vi "Ohmmeter.vi"() -> ()   [LabVIEW 2020]
uses:
  <vilib>/MakerHub/LINX/Private/Type Defs/LINX Ref.ctl
  <vilib>/MakerHub/LINX/Private/Type Defs/Platform.ctl
  <vilib>/MakerHub/LINX/Private/Type Defs/Interface.ctl
  <vilib>/MakerHub/LINX/Private/Device/Type Defs/LINX Device Config.ctl
  <vilib>/MakerHub/LINX/Private/Device/Type Defs/TCP Config.ctl
  <vilib>/MakerHub/LINX/Private/Device/Type Defs/Channels.ctl
  <vilib>/MakerHub/LINX/Public/Peripherals/Analog/Analog Read 1 Chan.vi
  <vilib>/MakerHub/LINX/Public/Peripherals/Analog/Analog Read N Chans.vi
  <vilib>/MakerHub/LINX/Private/Local IO/LinxAnalogRead.vi
  <vilib>/MakerHub/LINX/Public/Utilities/Check Channel.vi
  <vilib>/MakerHub/LINX/Public/Utilities/Open Serial.vi
  <vilib>/MakerHub/LINX/Private/Utilties/Generate Error.vi
  <vilib>/MakerHub/LINX/LMH-LINX.lvlib
  <vilib>/MakerHub/LINX/Private/Device/Device.lvlib
panel:
  in  "Tab Control":enum32{"Serial Com.", "Circuit", "Readings"}(tab)
  in  "Serial Port":refnum<visa-resource-name>="N/A"
  out "Connected?":bool
  in  "Start Serial Communication":bool
  in  "Stop Serial \nCommunication":bool
  out "Device Name":string
  out "2D Picture":picture
  in  "Ohmmeter Circuit\nParameters":T1
  in  "Read Data":bool
  in  "Pause Readings":bool
  in  "Save Data":bool
  out "Data History":dbl(graph)
  out "Reading?":bool
  in  "Read Freq. (Hz)":dbl
  in  "Stop Application":bool
  # "Serial Ohmmeter V.I."
  # "Serial  Communication"
  # "Communication State"
  # "Circuit  Parameters"
  # "Circuit Schematics"
  # "Readings State"
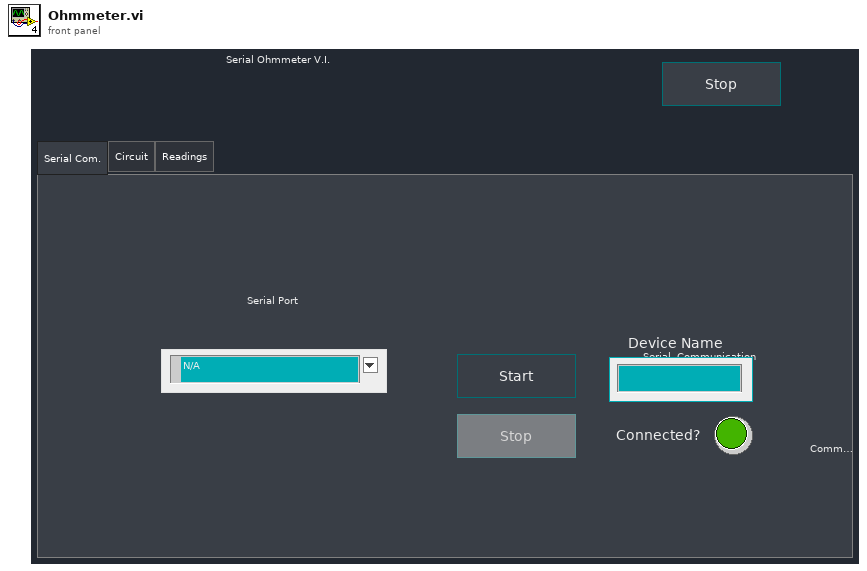
[diagram p1: front panel]
types:
  T1 = cluster{" Circuit Total Voltage (V)":dbl, " Reference Resistor (W)":dbl, "Analog Pin":u8}
  T2 = typedef "LMH-LINX.lvlib/LINX Ref.ctl" = cluster{"IO":T3, "Interface":T4, "LINX Device Config":T5}
  T3 = typedef "LMH-LINX.lvlib/Platform.ctl" = enum16{"Remote", "Local"}
  T4 = typedef "LMH-LINX.lvlib/Interface.ctl" = enum16{"Serial", "TCP"}
  T5 = typedef "LMH-LINX.lvlib/Device.lvlib/LINX Device Config.ctl" = cluster{"Interface":T4, "COM Port":refnum<visa-resource-name>, "TCP Configuration":T6, "Device Family":u8, "Device ID":u8, "Device Name":string, "TCP Ref":refnum<k5>, "Channels":T7}
  T6 = typedef "LMH-LINX.lvlib/Device.lvlib/TCP Config.ctl" = cluster{"IP Address":string, "Port":u16}
  T7 = typedef "LMH-LINX.lvlib/Channels.ctl" = cluster{"DI":u8[], "DO":u8[], "AI":u8[], "AO":u8[], "PWM":u8[], "QE":u8[], "UART":u8[], "I2C 2":u8[], "SPI":u8[], "CAN":u8[], "Servo":u8[], "AI Ref (V)":dbl, "AI Resolution (Bits)":u8, "AO Ref (V)":dbl, "AO Resolution (Bits)":u8}
  T8 = enum8{"Enabled", "Disabled", "Disabled and Grayed Out"}
  T9 = typedef "imagedata.ctl" = cluster{"image type":i32, "image depth":i32, "image":u8[], "mask":u8[], "colors":u32[], "Rectangle":cluster{"left":i16, "top":i16, "right":i16, "bottom":i16}}
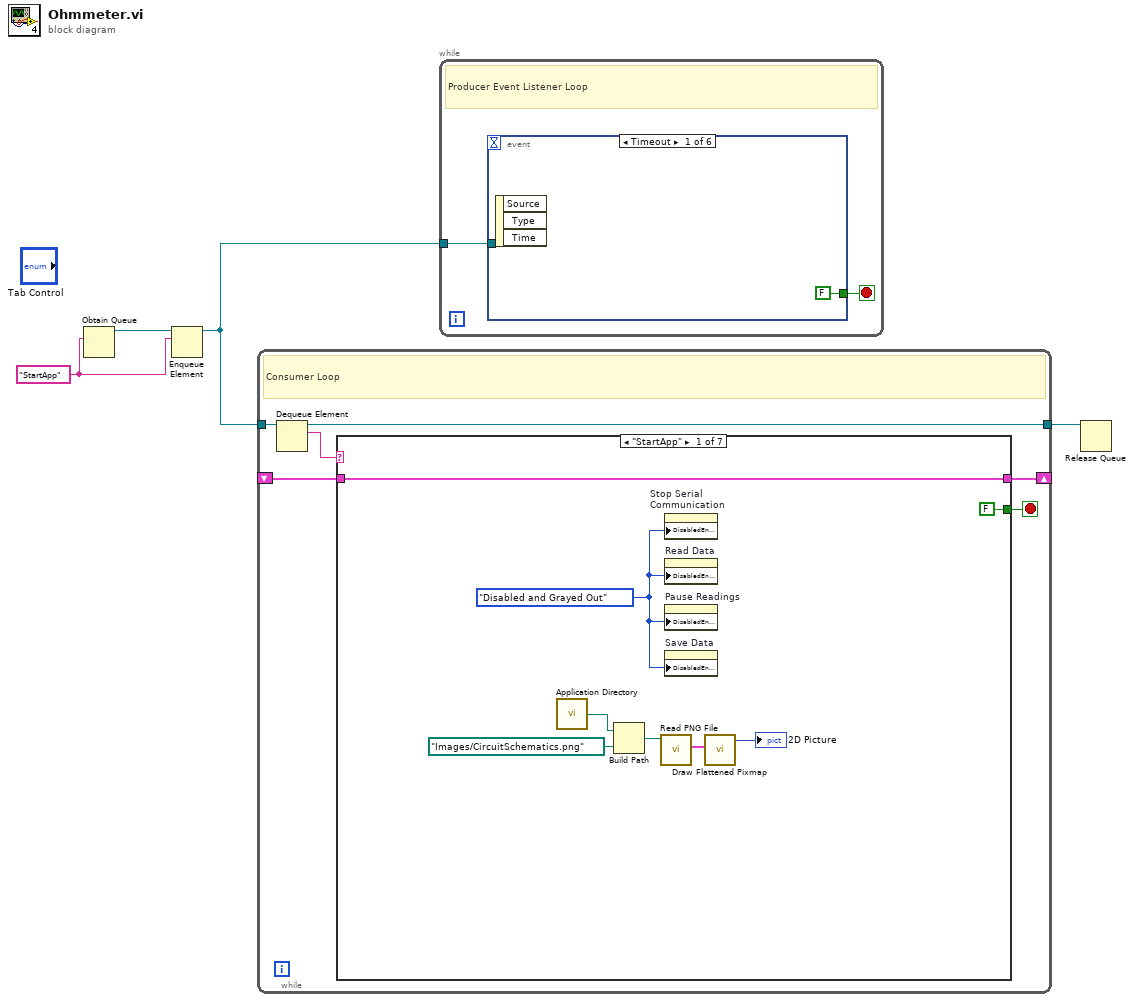
[diagram p0: block diagram]
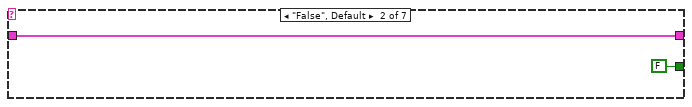
[diagram p2: hidden frame]
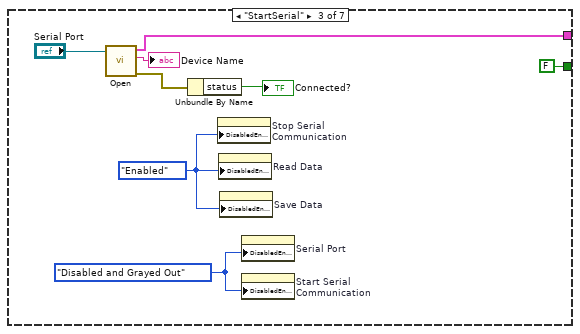
[diagram p3: hidden frame]
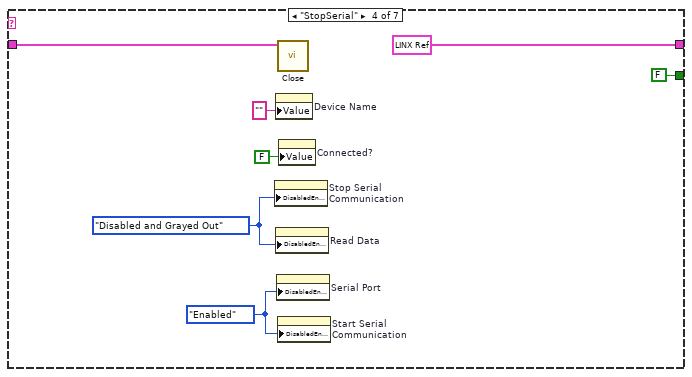
[diagram p4: hidden frame]
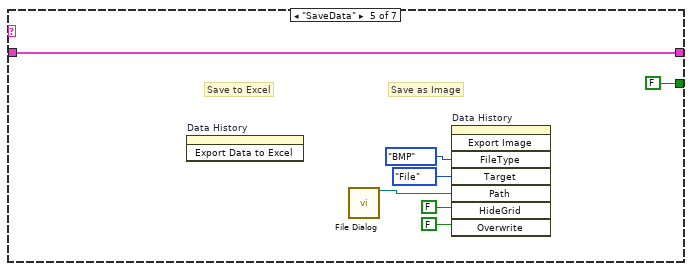
[diagram p5: hidden frame]
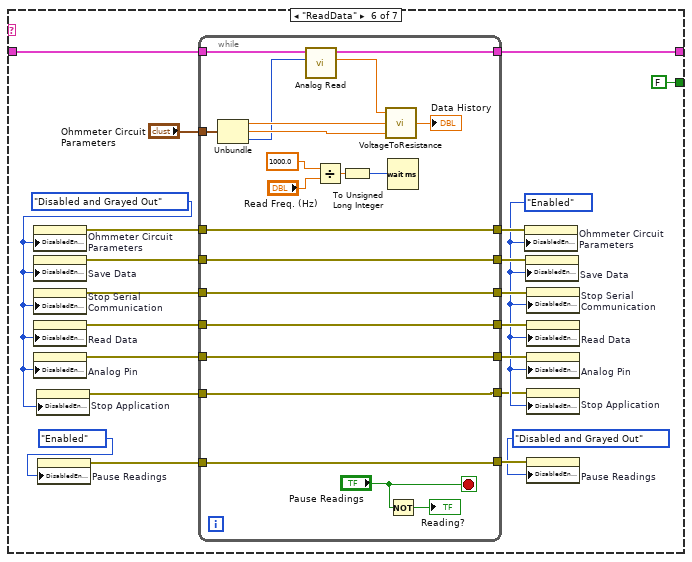
[diagram p6: hidden frame]
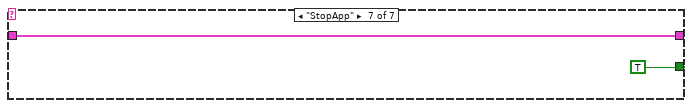
[diagram p7: hidden frame]
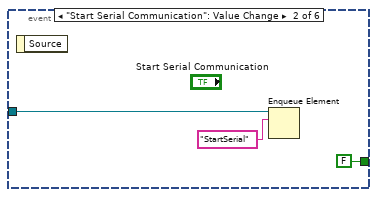
[diagram p8: hidden frame]
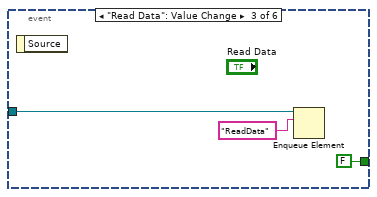
[diagram p9: hidden frame]
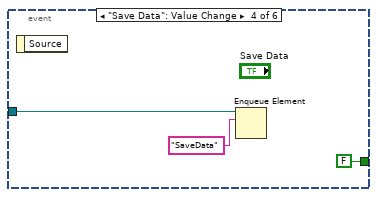
[diagram p10: hidden frame]
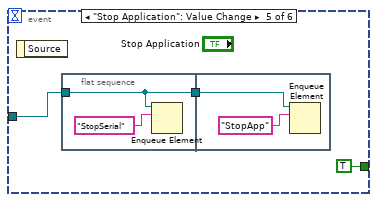
[diagram p11: hidden frame]
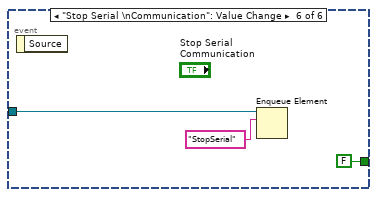
[diagram p12: hidden frame]
diagram:
  w1 = "StartApp"
  n1 = Obtain Queue(element data type=w1) -> (queue out=w2:refnum<queue>)  [unwired: 4 in, 2 out]
  n2 = Enqueue Element(queue=w2, element=w1) -> (queue out=w3:refnum<queue>)  [unwired: 2 in, 2 out]
  n3 = while {
    tunnel: w3 -> [w10]
    tunnel: [w7] -> w4
    shift-right: [w6] -> _
    shift-left: _ -> [w5]
    stop <- w8 stop-if-true
    # "Consumer Loop"
    n4 = Dequeue Element(queue=w10) -> (queue out=w7:refnum<queue>, element=w9:string)  [unwired: 2 in, 2 out]
    n5 = case shown="\"StartApp\"" w9 {
      tunnel: [FALSE FALSE FALSE FALSE FALSE FALSE TRUE] -> w8
      tunnel: [w16 w20 w26 T2 {"IO"=enum."Remote", "Interface"=enum."Serial", "LINX Device Config"={"Interface"=enum."Serial", "COM Port"="", "TCP Configuration"={"IP Address"="", "Port"=0}, "Device Family"=0, "Device ID"=0, "Device Name"="", "TCP Ref"=refnum, "Channels"={"DI"=[], "DO"=[], "AI"=[], "AO"=[], "PWM"=[], "QE"=[], "UART"=[], "I2C 2"=[], "SPI"=[], "CAN"=[], "Servo"=[], "AI Ref (V)"=0.0, "AI Resolution (Bits)"=0, "AO Ref (V)"=0.0, "AO Resolution (Bits)"=0}}} ("LINX Resource") w36 w62 w86] -> w6
      tunnel: w5 -> [w16 w20 _ w35 w36 w64 w86]
      frame "StartApp" {
        w18 = T8."Disabled and Grayed Out" ("Disabled")
        n6 = call <vilib>:"Application Directory.vi"() -> ("Application Directory"=w11:path)
        n7 = Build Path(base path=w11, name or relative path=path "Images/CircuitSchematics.png") -> (appended path=w14:path)
        n8 = call <vilib>:"Read PNG File.vi"("path to PNG file"=w14) -> ("image data"=w13:T9)  [unwired: 8 in, 2 out]
        n9 = property on="Stop Serial \nCommunication" class="Bool"("DisabledEnum"=w18) -> ()  [unwired: 2 in, 2 out]
        n10 = property on="Read Data" class="Bool"("DisabledEnum"=w18) -> ()  [unwired: 2 in, 2 out]
        n11 = property on="Pause Readings" class="Bool"("DisabledEnum"=w18) -> ()  [unwired: 2 in, 2 out]
        n12 = property on="Save Data" class="Bool"("DisabledEnum"=w18) -> ()  [unwired: 2 in, 2 out]
        n13 = call <vilib>:"Draw Flattened Pixmap.vi"("image data"=w13) -> ("new picture"=→"2D Picture":picture)  [unwired: 8 in]
      }
      frame "False", Default {
      }
      frame "StartSerial" {
        w22 = T8."Disabled and Grayed Out" ("Disabled")
        w23 = T8."Enabled" ("Disabled")
        n14 = call-poly <vilib>:"Open.vi"("Serial Port"="Serial Port") -> ("Error Out"=w25:errorcluster, "Device Name"=→"Device Name":string, "LINX Resource"=w26:T2)  [unwired: 8 in]
        n15 = Unbundle By Name(w25) -> ("status"=→"Connected?":bool)
        n16 = property on="Stop Serial \nCommunication" class="Bool"("DisabledEnum"=w23) -> ()  [unwired: 2 in, 2 out]
        n17 = property on="Read Data" class="Bool"("DisabledEnum"=w23) -> ()  [unwired: 2 in, 2 out]
        n18 = property on="Save Data" class="Bool"("DisabledEnum"=w23) -> ()  [unwired: 2 in, 2 out]
        n19 = property on="Serial Port" class="VISAName"("DisabledEnum"=w22) -> ()  [unwired: 2 in, 2 out]
        n20 = property on="Start Serial \nCommunication" class="Bool"("DisabledEnum"=w22) -> ()  [unwired: 2 in, 2 out]
      }
      frame "StopSerial" {
        w31 = T8."Enabled" ("Disabled")
        w30 = T8."Disabled and Grayed Out" ("Disabled")
        n21 = property on="Stop Serial \nCommunication" class="Bool"("DisabledEnum"=w30) -> ()  [unwired: 2 in, 2 out]
        n22 = property on="Device Name" class="Str"("Value"="" ("Device Name")) -> ()  [unwired: 2 in, 2 out]
        n23 = property on="Read Data" class="Bool"("DisabledEnum"=w30) -> ()  [unwired: 2 in, 2 out]
        n24 = property on="Serial Port" class="VISAName"("DisabledEnum"=w31) -> ()  [unwired: 2 in, 2 out]
        n25 = call <vilib>:"Close.vi"("LINX Resource"=w35) -> ()  [unwired: 10 in, 1 out]
        n26 = property on="Start Serial \nCommunication" class="Bool"("DisabledEnum"=w31) -> ()  [unwired: 2 in, 2 out]
        n27 = property on="Connected?" class="Bool (strict)"("Value"=FALSE ("Connected?")) -> ()  [unwired: 2 in, 2 out]
      }
      frame "SaveData" {
        # "Save as Image"
        # "Save to Excel"
        n28 = invoke on="Data History" class="WFChart (strict)" method="Export Data to Excel"() -> ()  [unwired: 3 in, 3 out]
        n29 = call "File Dialog"() -> ("selected path"=w39:path)  [unwired: 12 in, 3 out]
        n30 = invoke on="Data History" class="WFChart (strict)" method="Export Image"("FileType"=enum32{"BMP", "EPS", "EMF", "PICT"}."BMP" ("File Type"), "Target"=enum32{"File", "Clipboard"}."File", "Path"=w39, "HideGrid"=FALSE ("Hide Grid"), "Overwrite"=FALSE ("Always Overwrite")) -> ()  [unwired: 3 in, 8 out]
      }
      frame "ReadData" {
        w45 = T8."Enabled" ("Disabled")
        w46 = T8."Disabled and Grayed Out" ("Disabled")
        n31 = property on="Ohmmeter Circuit\nParameters" class="Clust (strict)"("DisabledEnum"=w46) -> (error out=w60:errorcluster)  [unwired: 2 in, 1 out]
        n32 = property on="Save Data" class="Bool"("DisabledEnum"=w46) -> (error out=w59:errorcluster)  [unwired: 2 in, 1 out]
        n33 = property on="Stop Serial \nCommunication" class="Bool"("DisabledEnum"=w46) -> (error out=w58:errorcluster)  [unwired: 2 in, 1 out]
        n34 = property on="Read Data" class="Bool"("DisabledEnum"=w46) -> (error out=w57:errorcluster)  [unwired: 2 in, 1 out]
        n35 = property on="Analog Pin" class="DigNum (strict)"("DisabledEnum"=w46) -> (error out=w56:errorcluster)  [unwired: 2 in, 1 out]
        n36 = property on="Stop Application" class="Bool"("DisabledEnum"=w46) -> (error out=w43:errorcluster)  [unwired: 2 in, 1 out]
        n37 = property on="Pause Readings" class="Bool"("DisabledEnum"=T8."Enabled" ("Disabled")) -> (error out=w55:errorcluster)  [unwired: 2 in, 1 out]
        n38 = while {
          tunnel: w64 -> [w85]
          tunnel: "Ohmmeter Circuit\nParameters" -> [w84]
          tunnel: [w83] -> w62
          tunnel: [w75] -> w54
          tunnel: w60 -> [w75]
          tunnel: [w74] -> w53
          tunnel: w59 -> [w74]
          tunnel: [w73] -> w52
          tunnel: w58 -> [w73]
          tunnel: [w72] -> w51
          tunnel: w57 -> [w72]
          tunnel: [w71] -> w50
          tunnel: w56 -> [w71]
          tunnel: [w70] -> w49
          tunnel: w55 -> [w70]
          tunnel: [w67] -> w44
          tunnel: w43 -> [w67]
          stop <- "Pause Readings" stop-if-true
          n39 = Unbundle(w84) -> ("Circuit Total Voltage (V)"=w81:dbl, "Reference Resistor (W)"=w80:dbl, "Analog Pin"=w66:u8)
          n40 = call-poly <vilib>:"Analog Read.vi"("Analog Channel"=w66, "LINX Resource"=w85) -> ("Voltage"=w82:dbl, "LINX Resource"=w83:T2)  [unwired: 6 in, 2 out]
          n41 = Divide(x=1000.0, y="Read Freq. (Hz)") -> (x/y=w76:dbl)
          n42 = To Unsigned Long Integer(number=w76) -> (unsigned 32bit integer=w77:u32)
          n43 = call "VoltageToResistance.vi"("Reference Resistance (ohms)"=w80, "Circuit Total Voltage (V)"=w81, "Voltage Measured"=w82) -> ("Resistance Measured (ohms)"=→"Data History":dbl)
          n44 = Wait (ms)(milliseconds to wait=w77) -> ()  [unwired: 1 out]
          n45 = Not(x="Pause Readings") -> (.not. x?=→"Reading?":bool)
        }
        n46 = property on="Ohmmeter Circuit\nParameters" class="Clust (strict)"(error in=w54, "DisabledEnum"=w45) -> ()  [unwired: 1 in, 2 out]
        n47 = property on="Save Data" class="Bool"(error in=w53, "DisabledEnum"=w45) -> ()  [unwired: 1 in, 2 out]
        n48 = property on="Stop Serial \nCommunication" class="Bool"(error in=w52, "DisabledEnum"=w45) -> ()  [unwired: 1 in, 2 out]
        n49 = property on="Read Data" class="Bool"(error in=w51, "DisabledEnum"=w45) -> ()  [unwired: 1 in, 2 out]
        n50 = property on="Analog Pin" class="DigNum (strict)"(error in=w50, "DisabledEnum"=w45) -> ()  [unwired: 1 in, 2 out]
        n51 = property on="Stop Application" class="Bool"(error in=w44, "DisabledEnum"=w45) -> ()  [unwired: 1 in, 2 out]
        n52 = property on="Pause Readings" class="Bool"(error in=w49, "DisabledEnum"=T8."Disabled and Grayed Out" ("Disabled")) -> ()  [unwired: 1 in, 2 out]
      }
      frame "StopApp" {
      }
    }
  }
  n53 = while {
    tunnel: w3 -> [w89]
    stop <- w88 stop-if-true
    # "Producer Event Listener Loop"
    n54 = event shown="[0] Timeout" {
      selector: _ -> [_ _ _ _ _ _]
      dyn-events: _ -> [_ _ _ _ _ _]
      timeout: _ -> [_ _ _ _ _ _]
      tunnel: w89 -> [_ w93 w95 w98 w101 w108]
      tunnel: [FALSE ("Stop Application") FALSE ("Stop Application") FALSE ("Stop Application") FALSE ("Stop Application") TRUE ("Stop Application") FALSE ("Stop Application")] -> w88
      event Timeout {
        n55 = event-data() -> ()  [unwired: 1 in, 3 out]
      }
      event "Start Serial Communication": Value Change {
        n56 = event-data() -> ()  [unwired: 1 in, 1 out]
        n57 = Enqueue Element(queue=w93, element="StartSerial") -> ()  [unwired: 2 in, 3 out]
      }
      event "Read Data": Value Change {
        n58 = event-data() -> ()  [unwired: 1 in, 1 out]
        n59 = Enqueue Element(queue=w95, element="ReadData") -> ()  [unwired: 2 in, 3 out]
      }
      event "Save Data": Value Change {
        n60 = event-data() -> ()  [unwired: 1 in, 1 out]
        n61 = Enqueue Element(queue=w98, element="SaveData") -> ()  [unwired: 2 in, 3 out]
      }
      event "Stop Application": Value Change {
        n62 = event-data() -> ()  [unwired: 1 in, 1 out]
        n63 = flat-sequence {
          tunnel: w101 -> [w103]
          tunnel: [w103] -> w100
          tunnel: w100 -> [w105]
          frame #0 {
            n64 = Enqueue Element(queue=w103, element="StopSerial") -> ()  [unwired: 2 in, 3 out]
          }
          frame #1 {
            n65 = Enqueue Element(queue=w105, element="StopApp") -> ()  [unwired: 2 in, 3 out]
          }
        }
      }
      event "Stop Serial \nCommunication": Value Change {
        n66 = event-data() -> ()  [unwired: 1 in, 1 out]
        n67 = Enqueue Element(queue=w108, element="StopSerial") -> ()  [unwired: 2 in, 3 out]
      }
    }
  }
  n68 = Release Queue(queue=w4) -> ()  [unwired: 2 in, 3 out]
